vi "CH_LM CallChain.vi"() -> (0 "ChallChain":string)   [LabVIEW 2012, in "CH_LM.lvlib"]
doc: "This VI retruns the VI call chain as string, excluding itself, to be used as input for the error cluster."
uses:
  CH_LM.lvlib
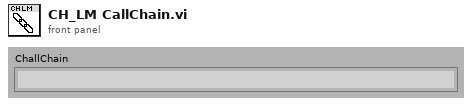
[diagram p1: front panel]
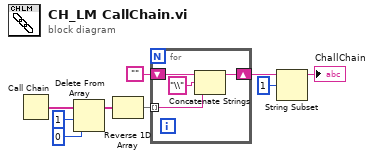
[diagram p0: block diagram]
diagram:
  n1 = Call Chain() -> (call chain=w8:string[])
  n2 = Delete From Array(array=w8, length=1, index=0) -> (array with subset deleted=w5:string[])  [unwired: 1 out]
  n3 = Reverse 1D Array(array=w5) -> (reversed array=w4:string[])
  n4 = for {
    shift-right: [w10] -> w3
    shift-left: "" ("Empty String Constant") -> [w13]
    tunnel: w4 -> [w11] mode=indexing
    n5 = Concatenate Strings(w13, "\\" ("string"), w11) -> (w10:string)
  }
  n6 = String Subset(string=w3, offset (0)=1) -> (substring=→"ChallChain":string)  [unwired: 1 out]
